vi "Read.vi"(7 "Map id":i32, 8 "Error In":errorcluster, 10 "Data in":dbl[](array[numeric]), 11 "Indices in":i32[](array[numeric])) -> (0 "Error Out":errorcluster, 2 "Data out":dbl[](array[numeric]), 3 "Indices out":i32[](array[numeric]))   [LabVIEW 2018]
uses:
  SharedMemoryTest.dll
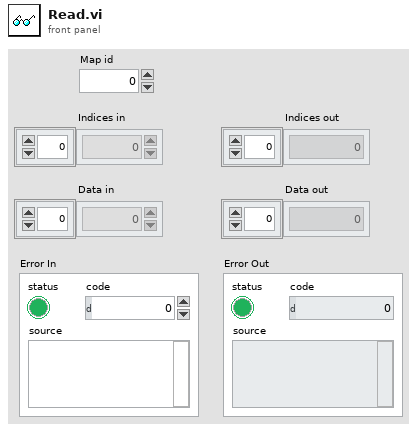
[diagram p1: front panel]
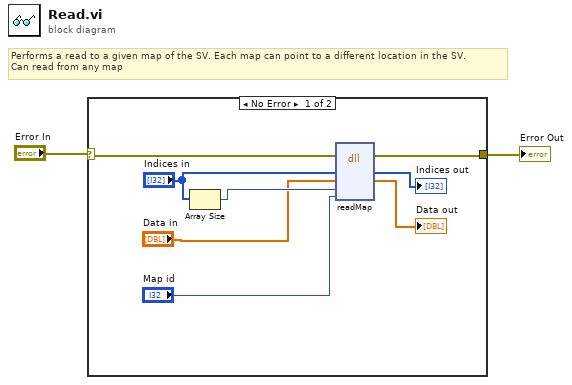
[diagram p0: block diagram]
diagram:
  # "Performs a read to a given map of the SV. Each map can point to a different location in the SV.\nCan read from any map"
  n1 = case shown="No Error" "Error In" {
    selector: "Error In" -> [w10 w11]
    tunnel: [w9 w11] -> w1
    frame No Error {
      n2 = Array Size(array="Indices in") -> (size(s)=w7:i32)
      n3 = dll-call lib="C:/Users/jaros/Desktop/UIF_StateVector/SV operations/SharedMemoryTest.dll" fn="readMap"(error in=w10, "idx"="Indices in", "data"="Data in", "length"=w7, "map id"="Map id") -> (error out=w9:errorcluster, "idx"=→"Indices out":i32[], "data"=→"Data out":dbl[])  [unwired: 5 in, 1 out]
    }
    frame Error {
    }
  }
  "Error Out" <- w1
